vi "FTW-JSON-CodeGen-GetTerms4.vi"(0 "State In":T2, 5 "XRef":refnum<vi>) -> (4 "Terms":T1(array[cluster]))   [LabVIEW 2012, in "FTW-JSON-Deserialize.xnode"]
uses:
  src/JSON/FTW-JSON-Deserialize.xnode
  FTW-JSON-CodeGen-State.ctl
panel:
  # "Inputs"
  # "Outputs"
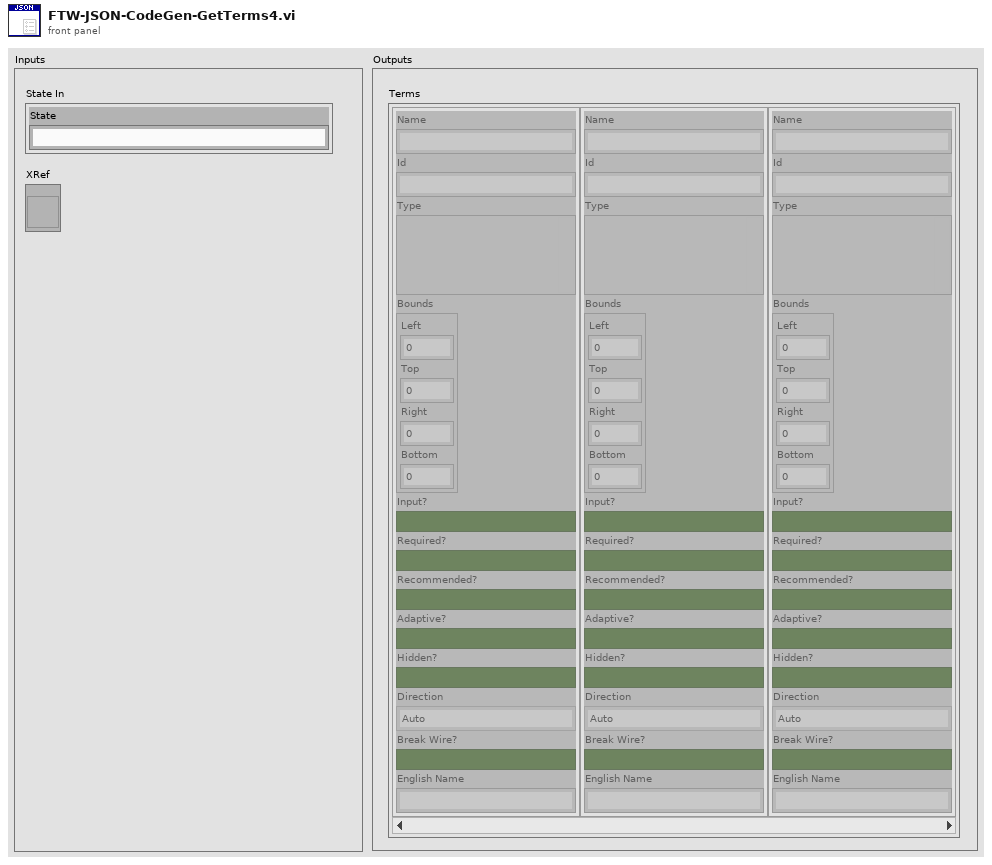
[diagram p1: front panel]
types:
  T1 = cluster{"Name":string, "Id":string, "Type":variant, "Bounds":cluster{"Left":i32, "Top":i32, "Right":i32, "Bottom":i32}, "Input?":bool, "Required?":bool, "Recommended?":bool, "Adaptive?":bool, "Hidden?":bool, "Direction":enum32{"Auto", "Up", "Down", "Left", "Right", "Center"}, "Break Wire?":bool, "English Name":string}[]
  T2 = typedef "FTW-JSON-Deserialize.xnode/FTW-JSON-CodeGen-State.ctl" = cluster{"State":string}
  T3 = cluster{"Name":string, "Id":string, "Type":variant, "Bounds":cluster{"Left":i32, "Top":i32, "Right":i32, "Bottom":i32}, "Input?":bool, "Required?":bool, "Recommended?":bool, "Adaptive?":bool, "Hidden?":bool, "Direction":enum32{"Auto", "Up", "Down", "Left", "Right", "Center"}, "Break Wire?":bool, "English Name":string}
  T4 = typedef "LVRectTypeDef.ctl" = cluster{"Left":i16, "Top":i16, "Right":i16, "Bottom":i16}
  T5 = enum16{"Invalid Wire Rule", "Required", "Recommended", "Optional", "Dynamic Dispatch"}[]
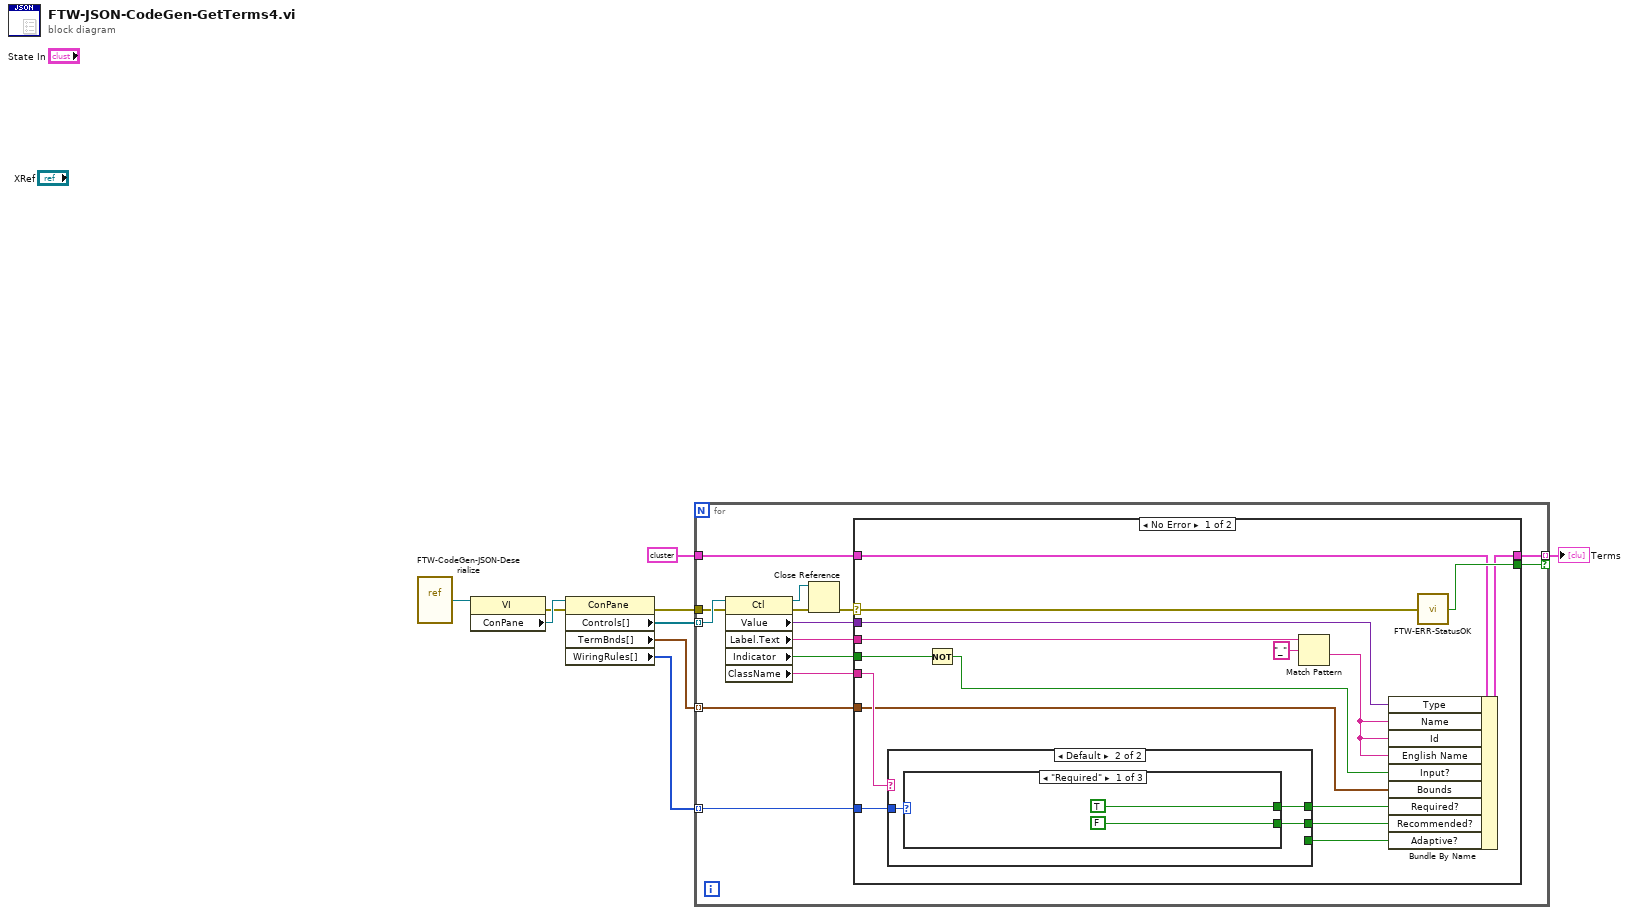
[diagram p0: block diagram]
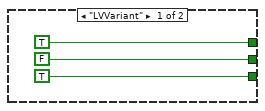
[diagram p2: hidden frame]
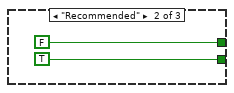
[diagram p3: hidden frame]
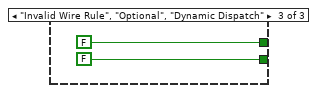
[diagram p4: hidden frame]
diagram:
  n1 = vi-ref "FTW-CodeGen-JSON-Deserialize.vi"() -> (w9:refnum<vi>)
  n2 = property class="VI"(reference=w9) -> (error out=w5:errorcluster, "ConPane"=w8:refnum<vi>)  [unwired: 1 in, 1 out]
  n3 = property class="ConPane"(reference=w8, error in=w5) -> (error out=w4:errorcluster, "Controls[]"=w7:refnum<vi>[], "TermBnds[]"=w3:T4[], "WiringRules[]"=w1:T5)  [unwired: 1 out]
  n4 = for {
    tunnel: w3 -> [w21] mode=indexing
    tunnel: w7 -> [w19] mode=indexing
    tunnel: w1 -> [w20] mode=indexing
    tunnel: T3 {"Name"="", "Id"="", "Type"=variant, "Bounds"={"Left"=0, "Top"=0, "Right"=0, "Bottom"=0}, "Input?"=FALSE, "Required?"=FALSE, "Recommended?"=FALSE, "Adaptive?"=FALSE, "Hidden?"=FALSE, "Direction"=enum."Auto", "Break Wire?"=FALSE, "English Name"=""} ("Term 4") -> [w23]
    tunnel: [w22] -> w6 mode=indexing if=w13
    tunnel: w4 -> [w14]
    n5 = property class="Ctl"(reference=w19, error in=w14) -> (reference out=w12:refnum<vi>, error out=w11:errorcluster, "Value"=w18:variant, "Label.Text"=w17:string, "Indicator"=w15:bool, "ClassName"=w16:string)
    n6 = Close Reference(reference=w12, error in (no error)=w11) -> (error out=w10:errorcluster)
    n7 = case shown="No Error" w10 {
      selector: w10 -> [w26 _]
      tunnel: w23 -> [w38 w52]
      tunnel: [w37 w52] -> w22
      tunnel: w21 -> [w25 _]
      tunnel: w20 -> [w36 _]
      tunnel: w18 -> [w33 _]
      tunnel: w16 -> [w32 _]
      tunnel: w17 -> [w29 _]
      tunnel: w15 -> [w30 _]
      tunnel: [w39 _] -> w13
      frame No Error {
        n8 = case shown="Default" w32 {
          tunnel: w36 -> [_ w45]
          tunnel: [TRUE w44] -> w35
          tunnel: [FALSE w43] -> w34
          tunnel: [TRUE _] -> w31
          frame "LVVariant" {
          }
          frame Default {
            n9 = case shown="\"Required\"" w45 {
              tunnel: [TRUE FALSE FALSE] -> w44
              tunnel: [FALSE TRUE FALSE] -> w43
              frame "Required" {
              }
              frame "Recommended" {
              }
              frame "Invalid Wire Rule", "Optional", "Dynamic Dispatch" {
              }
            }
          }
        }
        n10 = Not(x=w30) -> (.not. x?=w24:bool)
        n11 = Match Pattern(string=w29, regular expression="_") -> (after substring=w27:string)  [unwired: 1 in, 3 out]
        n12 = Bundle By Name(cluster=w38, "Type"=w33, "Name"=w27, "Id"=w27, "English Name"=w27, "Input?"=w24, "Bounds"=w25, "Required?"=w35, "Recommended?"=w34, "Adaptive?"=w31) -> (w37:T3)
        n13 = call "FTW-ERR-StatusOK.vi"("error to check"=w26) -> ("Status OK?"=w39:bool)
      }
      frame Error {
      }
    }
  }
  "Terms" <- w6
